vi "ke37xx Digital I-O Trigger Control.vi"(0 "VISA Resource Name":refnum<visa-resource-name>, 5 "Action (0: Clear)":enum16{"Clear", "Wait", "Assert", "Release"}(ring), 7 "Line (1)":u8=1 min=1 max=14, 9 "Timeout Seconds (2 sec)":dbl=2.0, 11 "error in (no error)":errorcluster) -> (4 "VISA Resource Name Out":refnum<visa-resource-name>, 8 "Triggered":bool, 15 "error out":errorcluster)   [LabVIEW 2009, in "Keithley 3700 Series.lvlib"]
doc: "This VI allows you to control the digital I/O triggering system. You can assert, release, or clear a specific digital I/O trigger line. You can also wait for a specific digital I/O line event detector to enter the detected state."
uses:
  <instrlib>/Keithley 3706/Keithley 3700 Series.lvlib
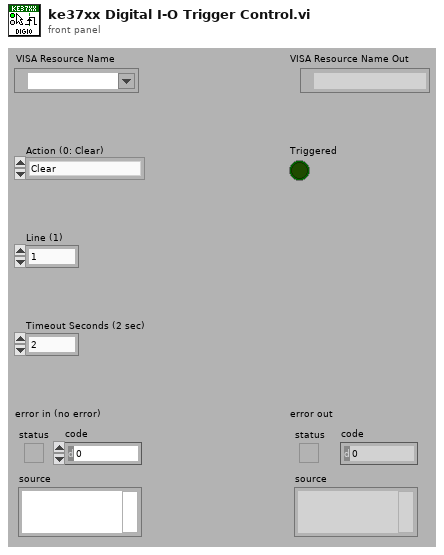
[diagram p1: front panel]
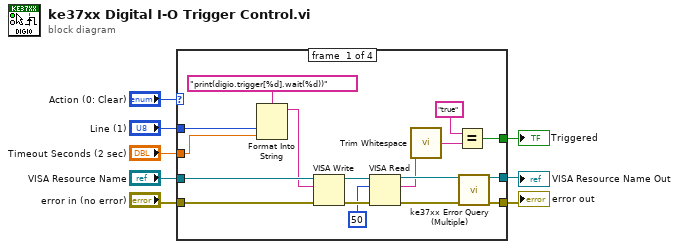
[diagram p0: block diagram]
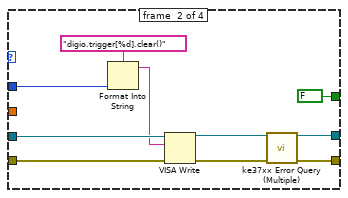
[diagram p2: hidden frame]
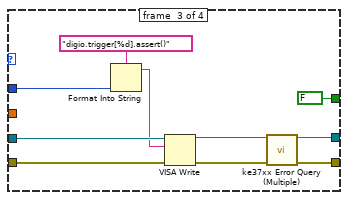
[diagram p3: hidden frame]
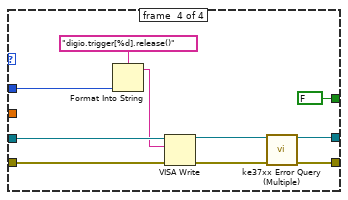
[diagram p4: hidden frame]
diagram:
  n1 = case shown="\"Wait\"" "Action (0: Clear)" {
    tunnel: [w25 w35 w45 w55] -> w8
    tunnel: [w24 w34 w44 w54] -> w7
    tunnel: "VISA Resource Name" -> [w23 w33 w43 w53]
    tunnel: "error in (no error)" -> [w22 w32 w42 w52]
    tunnel: "Line (1)" -> [w15 w31 w40 w50]
    tunnel: "Timeout Seconds (2 sec)" -> [w14 _ _ _]
    tunnel: [w9 FALSE FALSE FALSE] -> w1
    frame #0 {
      n2 = Format Into String(format string="print(digio.trigger[%d].wait(%d))", w15, w14) -> (resulting string=w13:string)  [unwired: 2 in, 1 out]
      n3 = VISA Write(VISA resource name=w23, write buffer=w13, error in (no error)=w22) -> (VISA resource name out=w20:refnum<visa-resource-name>, error out=w21:errorcluster)  [unwired: 1 out]
      n4 = VISA Read(VISA resource name=w20, byte count=u32 50, error in (no error)=w21) -> (VISA resource name out=w19:refnum<visa-resource-name>, read buffer=w12:string, error out=w18:errorcluster)  [unwired: 1 out]
      n5 = call <vilib>:"Trim Whitespace.vi"("string"=w12) -> ("trimmed string"=w11:string)  [unwired: 1 in]
      n6 = Equal?(x="true", y=w11) -> (x = y?=w9:bool)
      n7 = call <instrlib>:"ke37xx Error Query (Multiple).vi"("VISA resource name"=w19, "error in (no error)"=w18) -> ("VISA resource name out"=w25:refnum<visa-resource-name>, "error out"=w24:errorcluster)  [unwired: 12 out]
    }
    frame #1 {
      n8 = Format Into String(format string="digio.trigger[%d].clear()", w31) -> (resulting string=w30:string)  [unwired: 2 in, 1 out]
      n9 = VISA Write(VISA resource name=w33, write buffer=w30, error in (no error)=w32) -> (VISA resource name out=w29:refnum<visa-resource-name>, error out=w28:errorcluster)  [unwired: 1 out]
      n10 = call <instrlib>:"ke37xx Error Query (Multiple).vi"("VISA resource name"=w29, "error in (no error)"=w28) -> ("VISA resource name out"=w35:refnum<visa-resource-name>, "error out"=w34:errorcluster)  [unwired: 12 out]
    }
    frame #2 {
      n11 = Format Into String(format string="digio.trigger[%d].assert()", w40) -> (resulting string=w39:string)  [unwired: 2 in, 1 out]
      n12 = VISA Write(VISA resource name=w43, write buffer=w39, error in (no error)=w42) -> (VISA resource name out=w38:refnum<visa-resource-name>, error out=w37:errorcluster)  [unwired: 1 out]
      n13 = call <instrlib>:"ke37xx Error Query (Multiple).vi"("VISA resource name"=w38, "error in (no error)"=w37) -> ("VISA resource name out"=w45:refnum<visa-resource-name>, "error out"=w44:errorcluster)  [unwired: 12 out]
    }
    frame #3 {
      n14 = Format Into String(format string="digio.trigger[%d].release()", w50) -> (resulting string=w49:string)  [unwired: 2 in, 1 out]
      n15 = VISA Write(VISA resource name=w53, write buffer=w49, error in (no error)=w52) -> (VISA resource name out=w48:refnum<visa-resource-name>, error out=w47:errorcluster)  [unwired: 1 out]
      n16 = call <instrlib>:"ke37xx Error Query (Multiple).vi"("VISA resource name"=w48, "error in (no error)"=w47) -> ("VISA resource name out"=w55:refnum<visa-resource-name>, "error out"=w54:errorcluster)  [unwired: 12 out]
    }
  }
  "VISA Resource Name Out" <- w8
  "error out" <- w7
  "Triggered" <- w1
